vi "Local median of array from video.vi"(3 "Number of frames for median":i32, 4 "Read Frame Number":u32, 5 "Avi Refnum":T1) -> (1 "Local median array":u8[][](array[numeric]), 2 "Avi Refnum (duplicate)":T1)   [LabVIEW 2018]
uses:
  <vilib>/vision/Avi1.llb/AviRefnum.ctl
  <vilib>/Analysis/NI_AALBase.lvlib
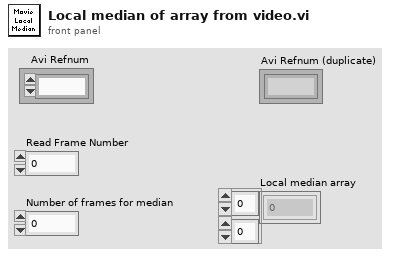
[diagram p1: front panel]
types:
  T1 = typedef "AviRefnum.ctl" = refnum<k1>
  T2 = cluster{"width":u32, "height":u32, "framesPerSecond":u32, "compressionFilter":string, "hasData":bool}
  T3 = typedef "IMAQ Image.ctl" = refnum<image>
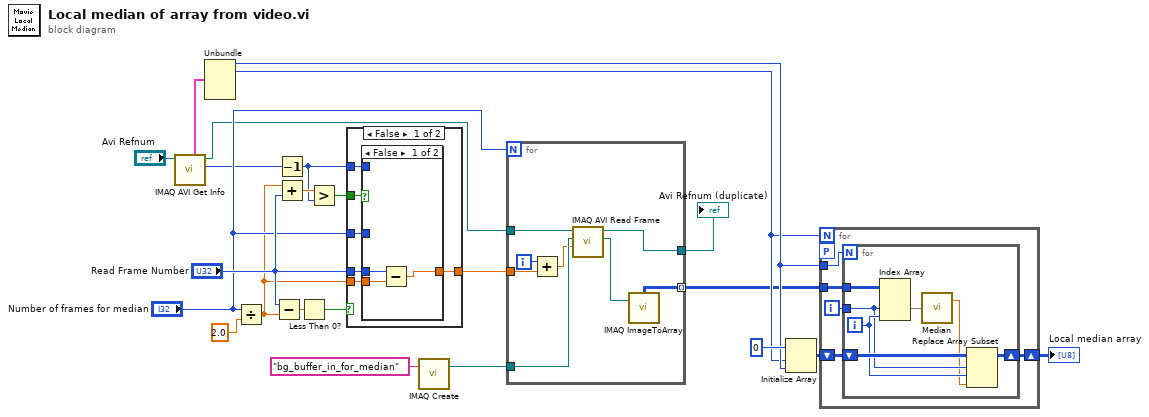
[diagram p0: block diagram]
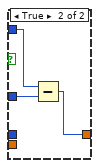
[diagram p2: hidden frame]
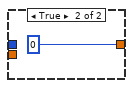
[diagram p3: hidden frame]
diagram:
  n1 = call "IMAQ AVI Get Info"("Avi Refnum"="Avi Refnum") -> ("Number of Frames"=w2:u32, "Avi Refnum (duplicate)"=w3:T1, "Frame Data"=w4:T2)  [unwired: 6 in, 2 out]
  n2 = Unbundle(w4) -> ("width"=w17:u32, "height"=w16:u32)  [unwired: 3 out]
  n3 = Divide(x="Number of frames for median", y=2.0) -> (x/y=w6:dbl)
  n4 = Subtract(x="Read Frame Number", y=w6) -> (x-y=w19:dbl)
  n5 = Decrement(x=w2) -> (x-1=w12:u32)
  n6 = Add(x=w6, y="Read Frame Number") -> (x+y=w14:dbl)
  n7 = Less Than 0?(x=w19) -> (x < 0?=w18:bool)
  n8 = Greater?(x=w14, y=w12) -> (0:w13:bool)
  n9 = case shown="False" w18 {
    tunnel: "Read Frame Number" -> [w28 _]
    tunnel: [w27 u32 0 ("Read Frame Number")] -> w10
    tunnel: w13 -> [w29 _]
    tunnel: w12 -> [w26 _]
    tunnel: "Number of frames for median" -> [w25 _]
    tunnel: w6 -> [w24 _]
    frame False {
      n10 = case shown="False" w29 {
        tunnel: w28 -> [w32 _]
        tunnel: [w31 w33] -> w27
        tunnel: w26 -> [_ w35]
        tunnel: w25 -> [_ w34]
        tunnel: w24 -> [w30 _]
        frame False {
          n11 = Subtract(x=w32, y=w30) -> (x-y=w31:dbl)
        }
        frame True {
          n12 = Subtract(x=w35, y=w34) -> (x-y=w33:u32)
        }
      }
    }
    frame True {
    }
  }
  n13 = call "IMAQ Create"("Image Name"="bg_buffer_in_for_median") -> ("New Image"=w8:T3)  [unwired: 4 in, 1 out]
  n14 = for {
    N: "Number of frames for median" -> [_]
    tunnel: w10 -> [w44]
    tunnel: w3 -> [w41]
    tunnel: w8 -> [w40]
    tunnel: [w37] -> w1
    tunnel: [w42] -> w7 mode=indexing
    i -> [w43]
    n15 = Add(x=w43, y=w44) -> (x+y=w39:dbl)
    n16 = call "IMAQ AVI Read Frame"("Frame Number"=w39, "Image"=w40, "Avi Refnum"=w41) -> ("Image Out"=w38:T3, "Avi Refnum (duplicate)"=w37:T1)  [unwired: 5 in, 2 out]
    n17 = call "IMAQ ImageToArray"("Image"=w38) -> ("Image Pixels (U8)"=w42:u8[][])  [unwired: 3 in, 4 out]
  }
  "Avi Refnum (duplicate)" <- w1
  n18 = Initialize Array(u8 0 ("element"), w16, w17) -> (w22:u8[][])
  n19 = for {
    N: w16 -> [_]
    tunnel: w17 -> [w49]
    shift-right: [w47] -> w21
    shift-left: w22 -> [w48]
    tunnel: w7 -> [w46]
    workers-P: _ -> [_]
    i -> [w45]
    n20 = for {
      N: w49 -> [_]
      shift-right: [w53] -> w47
      shift-left: w48 -> [w56]
      tunnel: w46 -> [w55]
      tunnel: w45 -> [w51]
      i -> [w52]
      n21 = Index Array(array=w55, index (dim 1)=w51, index (dim 2)=w52) -> (element=w54:u8[])  [unwired: 1 in]
      n22 = call <vilib>:"Median.vi"("X"=w54) -> ("median"=w50:dbl)  [unwired: 1 out]
      n23 = Replace Array Subset(array=w56, new element=w50, index (row)=w51, index (col)=w52) -> (w53:u8[][])
    }
  }
  "Local median array" <- w21
